vi "Cieślikiewicz1_1.vi"   [LabVIEW 2020]
types:
  T1 = typedef "Rendezvous RefNum" = refnum<k1>
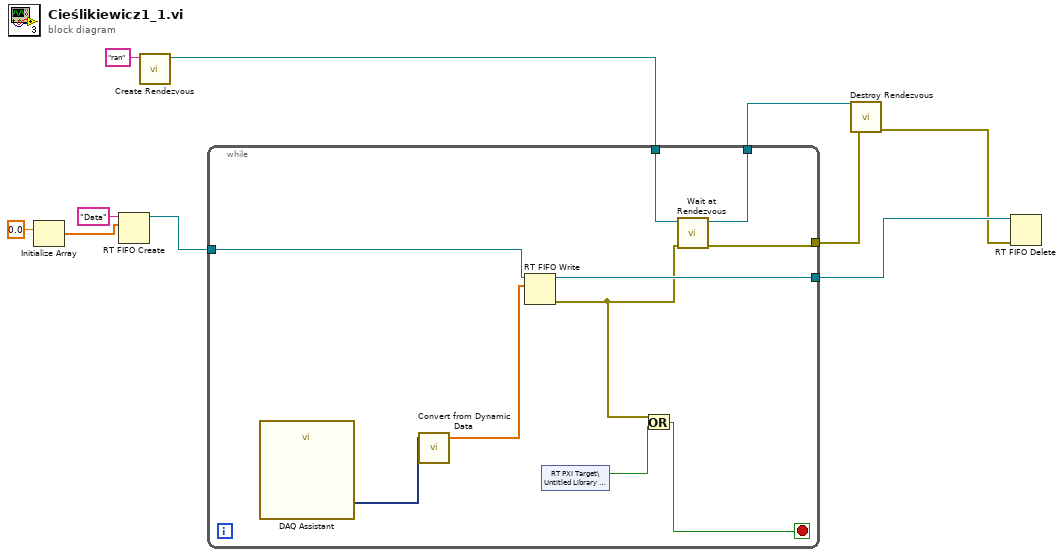
[diagram p0: block diagram]
diagram:
  n1 = Initialize Array(0.0 ("element")) -> (w8:dbl[])  [unwired: 1 in]
  n2 = RT FIFO Create(0:"Data" ("name (unnamed)"), 1:w8) -> (8:w6:refnum<k33>)  [unwired: 6 in, 2 out]
  n3 = call <vilib>:"Create Rendezvous.vi"("name (unnamed)"="ran") -> ("rendezvous"=w5:T1)  [unwired: 4 in, 2 out]
  n4 = while {
    tunnel: w6 -> [w20]
    tunnel: w5 -> [w18]
    tunnel: [w17] -> w4
    tunnel: [w16] -> w3
    tunnel: [w15] -> w2
    stop <- w14 stop-if-true
    n5 = call "DAQ Assistant"() -> ("data"=w11:dynamicdata)  [unwired: 17 in, 2 out]
    n6 = call "Convert from Dynamic Data"("Dynamic Data Type"=w11) -> ("Array"=w19:dbl[])  [unwired: 3 in]
    n7 = RT FIFO Write(0:w20, 1:w19) -> (8:w16:refnum<k33>, 11:w13:errorcluster)  [unwired: 3 in, 2 out]
    n8 = shared-variable "RT PXI Target\\Untitled Library 1.lvlib\\stop"() -> (w12:bool)  [unwired: 1 in, 1 out]
    n9 = Or(x=w13, y=w12) -> (x .or. y?=w14:bool)
    n10 = call <vilib>:"Wait at Rendezvous.vi"("error in (no error)"=w13, "rendezvous"=w18) -> ("error out"=w15:errorcluster, "rendezvous out"=w17:T1)  [unwired: 3 in, 1 out]
  }
  n11 = call <vilib>:"Destroy Rendezvous.vi"("error in (no error)"=w2, "rendezvous"=w4) -> ("error out"=w1:errorcluster)  [unwired: 4 in, 1 out]
  n12 = RT FIFO Delete(0:w3, 3:w1) -> ()  [unwired: 1 in, 1 out]
